vi "excelrowconcat_singlecol.vi"() -> ()   [LabVIEW 2020]
uses:
  <vilib>/addons/_office/excel.llb/Excel Get Data ([dbl]).vi
  <vilib>/Utility/file.llb/Write To Spreadsheet File (DBL).vi
  <vilib>/Utility/NIReport.llb/NI_report.lvclass
  <vilib>/Utility/NIReport.llb/Excel/NI_Excel.lvclass
  <vilib>/addons/_office/NI_ReportGenerationToolkit.lvlib
panel:
  out "LR Sheet Values":ext[][](array[numeric])=[[1.0, 16.0, 31.0, 46.0], [2.0, 17.0, 32.0, 47.0], [3.0, 18.0, 33.0, 48.0], [4.0, 19.0, 34.0, 49.0], [5.0, 20.0, 35.0, 50.0], [6.0, 21.0, 36.0, 51.0], [7.0, 22.0, 37.0, 52.0], [8.0, 23.0, 38.0, 53.0], [9.0, 24.0, 39.0, 54.0], [10.0, 25.0, 40.0, 55.0], [11.0, 26.0, 41.0, 56.0], [12.0, 27.0, 42.0, 57.0], [13.0, 28.0, 43.0, 58.0], [14.0, 29.0, 44.0, 59.0], [15.0, 30.0, 45.0, 60.0]] format="%_6e"
  out "Total LR Selected Row":i32=3
  in  "Tab Control":enum32{"HR", "LR"}(tab)
  out "LR Stack Col":ext[](array[numeric])=[1.0, 3.0, 5.0, 16.0, 18.0, 20.0, 31.0, 33.0, 35.0, 46.0, 48.0, 50.0] format="%#_6e"
  out "LR Added row":ext[][](array[numeric])=[[1.0, 16.0, 31.0, 46.0], [3.0, 18.0, 33.0, 48.0], [5.0, 20.0, 35.0, 50.0]] format="%#_6e"
  out "LR Selected Column":ext[](array[numeric])=[46.0, 48.0, 50.0] format="%#_6e"
  out "LR selected row":ext[](array[numeric])=[5.0, 20.0, 35.0, 50.0] format="%#_6e"
  in  "Low resgistananc state  Row Number (2,4,)":string="1,3,5"
  out "Columns":i32=4
  out "Rows":i32=15
  in  "Excel._Worksheet":refnum<k7>
  in  "Excel._Application":refnum<k7>
  out "HR Stack Col":ext[](array[numeric])=[1.0, 3.0, 5.0, 16.0, 18.0, 20.0, 31.0, 33.0, 35.0, 46.0, 48.0, 50.0] format="%#_6e"
  out "HR Selected Column":ext[](array[numeric])=[46.0, 48.0, 50.0] format="%#_6e"
  in  "precission":string="6"
  in  "Destination path for cutting rows":path=path "C:/Users/lab user/Desktop/cm/single column"
  in  "row cut file name (no extension)":string="saaaa"
  out "HR selected row":ext[](array[numeric])=[5.0, 20.0, 35.0, 50.0] format="%#_6e"
  in  "Hi resgistananc state  Row Number (1,3,)":string="1,3,5"
  out "Total HR Selected Row":i32=3
  in  "Select Excel file":path=path "C:/Users/lab user/Desktop/cm/single column/sc.xls"
  out "HR Added row":ext[][](array[numeric])=[[1.0, 16.0, 31.0, 46.0], [3.0, 18.0, 33.0, 48.0], [5.0, 20.0, 35.0, 50.0]] format="%#_6e"
  out "HR Sheet Values":ext[][](array[numeric])=[[1.0, 16.0, 31.0, 46.0], [2.0, 17.0, 32.0, 47.0], [3.0, 18.0, 33.0, 48.0], [4.0, 19.0, 34.0, 49.0], [5.0, 20.0, 35.0, 50.0], [6.0, 21.0, 36.0, 51.0], [7.0, 22.0, 37.0, 52.0], [8.0, 23.0, 38.0, 53.0], [9.0, 24.0, 39.0, 54.0], [10.0, 25.0, 40.0, 55.0], [11.0, 26.0, 41.0, 56.0], [12.0, 27.0, 42.0, 57.0], [13.0, 28.0, 43.0, 58.0], [14.0, 29.0, 44.0, 59.0], [15.0, 30.0, 45.0, 60.0]] format="%_6e"
  # "HR column stack output will be save in same directory\nrow cut file name_HR_single_col.xls"
  # "LR column stack output will be save in same directory\nrow cut file name_LR_single_col.xls"
  # "HR Row cut output will be save in same directory\nrow cut file name_HR.xls"
  # "LR Row cut  output will be save in same directory\nrow cut file name_LR.xls"
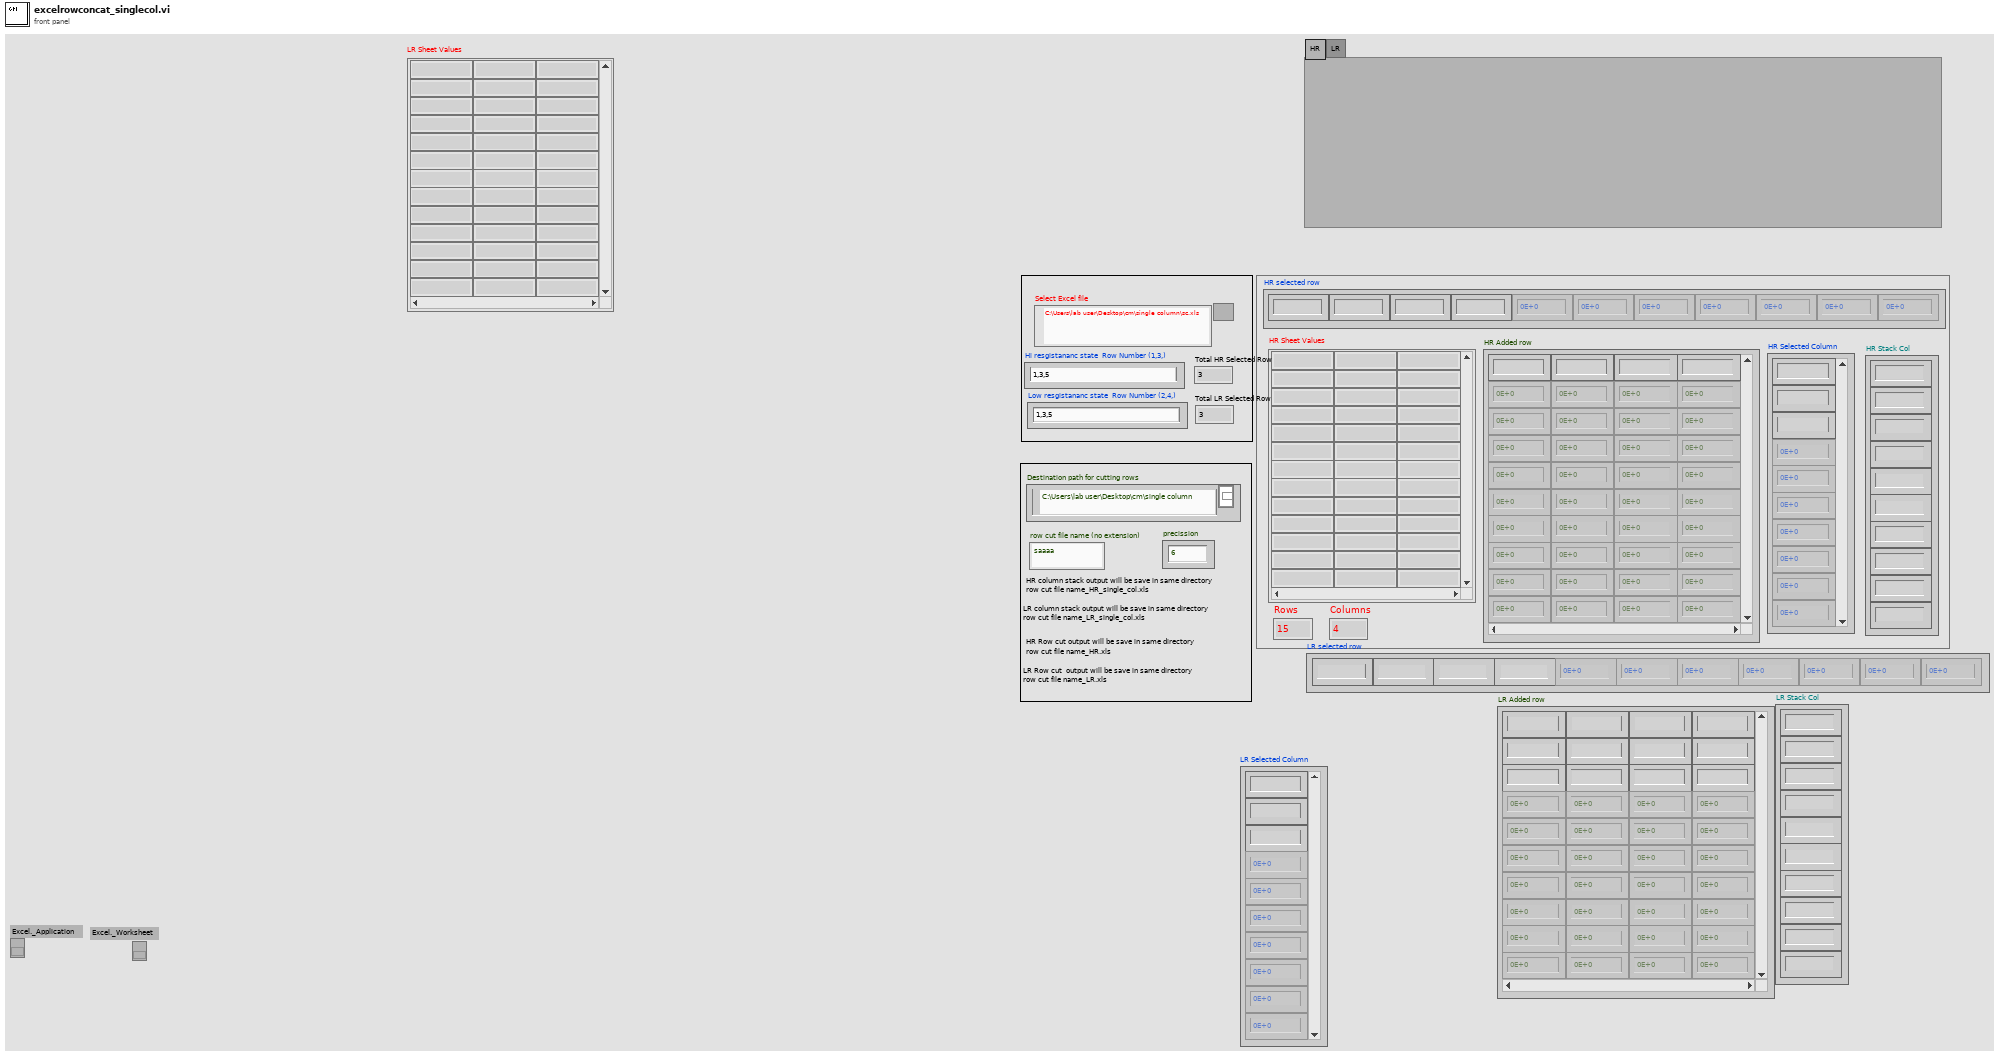
[diagram p1: front panel]
types:
  T1 = enum16{"Standard Report", "HTML", "Word", "Excel"}
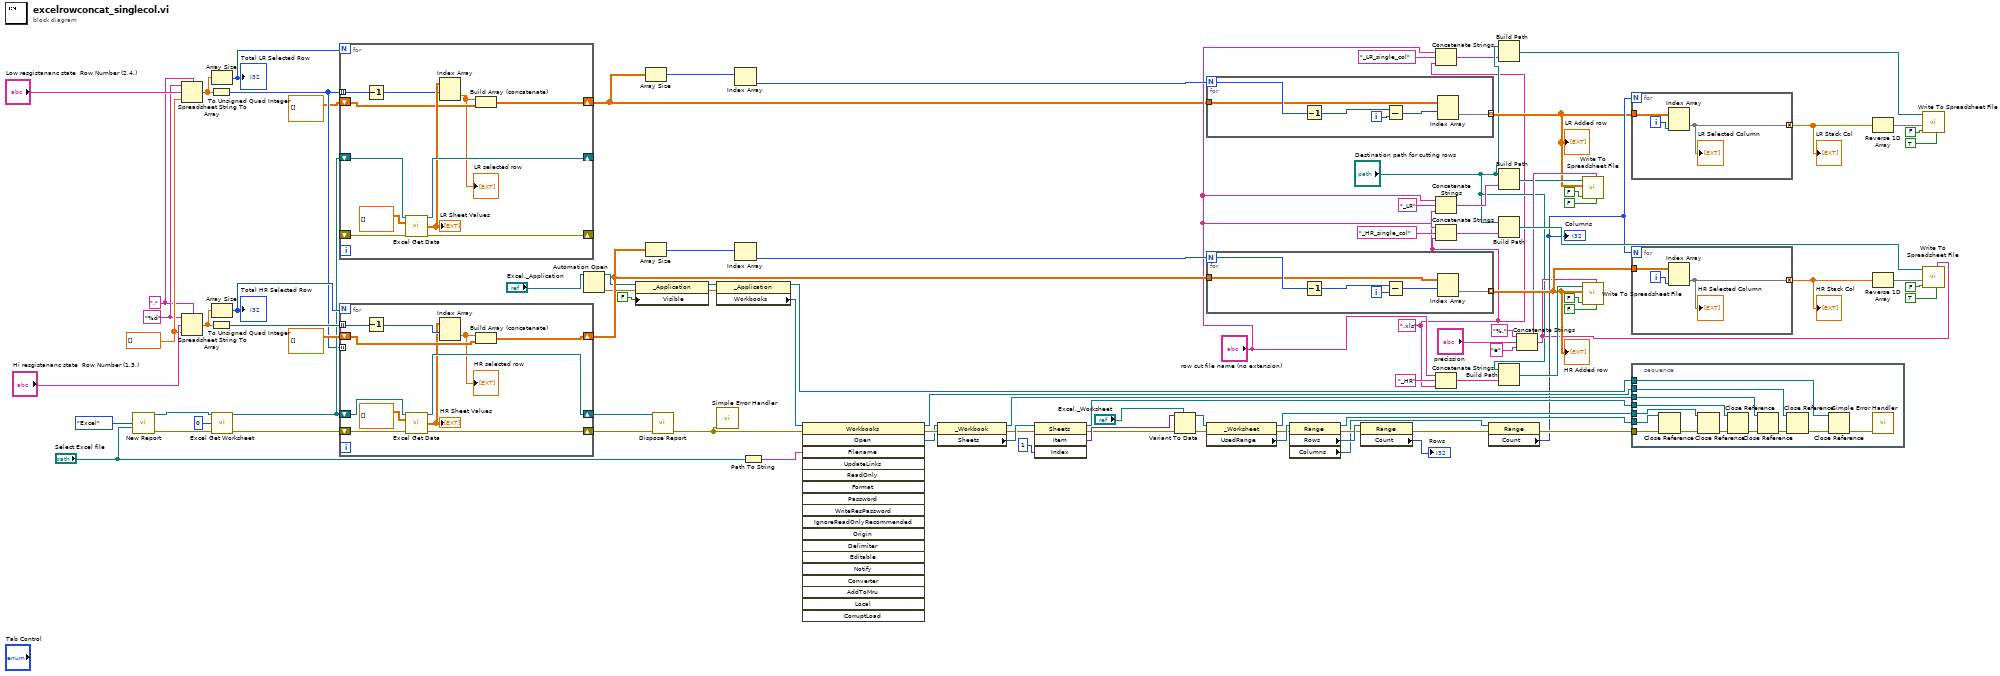
[diagram p0: block diagram]
diagram:
  w11 = ".xls" ("string")
  w32 = dbl[] []
  w29 = "," ("delimiter (Tab)")
  w30 = "%d" ("format string")
  n1 = call <vilib>:"New Report.vi"("report type"=T1."Excel", "template (empty)"="Select Excel file") -> ("report out"=w86:refnum<class "NI_report.lvclass">, "error out"=w87:errorcluster)  [unwired: 12 in]
  n2 = Spreadsheet String To Array(delimiter (Tab)=w29, format string=w30, spreadsheet string="Low resgistananc state  Row Number (2,4,)", array type (2D Dbl)=w32) -> (array=w6:dbl[])
  n3 = Spreadsheet String To Array(delimiter (Tab)=w29, format string=w30, spreadsheet string="Hi resgistananc state  Row Number (1,3,)", array type (2D Dbl)=w32) -> (array=w90:dbl[])
  n4 = To Unsigned Quad Integer(1:w6) -> (0:w4:u64[])
  n5 = To Unsigned Quad Integer(1:w90) -> (0:w89:u64[])
  n6 = Array Size(array=w6) -> (size(s)=w1:i32)
  "Total LR Selected Row" <- w1
  n7 = Array Size(array=w90) -> (size(s)=w69:i32)
  "Total HR Selected Row" <- w69
  n8 = call <vilib>:"Excel Get Worksheet.vi"("report in"=w86, "worksheet index (0)"=0, "error in (no error)"=w87) -> ("report out"=w5:refnum<class "NI_report.lvclass">, "error out"=w85:errorcluster)  [unwired: 11 in]
  n9 = for {
    N: w1 -> [_]
    shift-right: [w105] -> _
    shift-left: w5 -> [w102]
    shift-right: [w104] -> _
    shift-left: _ -> [w103]
    tunnel: w4 -> [w100] mode=indexing
    shift-right: [w98] -> w3
    shift-left: ext[][] [] -> [w97]
    n10 = Decrement(x=w100) -> (x-1=w99:u64)
    n11 = call-poly <vilib>:"Excel Get Data.vi"("report in"=w102, "data type"=ext[][] [], "error in (no error)"=w103) -> ("report out"=w105:refnum<class "NI_report.lvclass">, "data"=w101:ext[][], "error out"=w104:errorcluster)  [unwired: 10 in]
    "LR Sheet Values" <- w101
    n12 = Index Array(array=w101, index (row)=w99) -> (element=w96:ext[])  [unwired: 1 in]
    "LR selected row" <- w96
    n13 = Build Array (concatenate)(w96, w97) -> (w98:ext[][])
  }
  n14 = for {
    N: w69 -> [_]
    shift-right: [w116] -> w95
    shift-left: w5 -> [w111]
    shift-right: [w115] -> w94
    shift-left: w85 -> [w112]
    shift-right: [w113] -> w84
    shift-left: ext[][] [] -> [w114]
    tunnel: w89 -> [w110] mode=indexing
    tunnel: w4 -> [_] mode=indexing
    n15 = Decrement(x=w110) -> (x-1=w109:u64)
    n16 = call-poly <vilib>:"Excel Get Data.vi"("report in"=w111, "data type"=ext[][] [], "error in (no error)"=w112) -> ("report out"=w116:refnum<class "NI_report.lvclass">, "data"=w107:ext[][], "error out"=w115:errorcluster)  [unwired: 10 in]
    "HR Sheet Values" <- w107
    n17 = Index Array(array=w107, index (row)=w109) -> (element=w108:ext[])  [unwired: 1 in]
    "HR selected row" <- w108
    n18 = Build Array (concatenate)(w108, w114) -> (w113:ext[][])
  }
  n19 = Automation Open(Automation Refnum="Excel._Application") -> (Automation Refnum=w59:refnum<k7>, error out=w62:errorcluster)  [unwired: 3 in]
  n20 = property class="_Application"(reference=w59, error in=w62, "Visible"=FALSE ("Make Excel Visible")) -> (reference out=w58:refnum<k7>, error out=w61:errorcluster)
  n21 = Array Size(array=w3) -> (size(s)=w27:i32[])
  n22 = Array Size(array=w84) -> (size(s)=w82:i32[])
  n23 = call-dynamic "Dispose Report.vi"("report in"=w95, "error in (no error)"=w94) -> ("error out"=w35:errorcluster)  [unwired: 13 in]
  n24 = property class="_Application"(reference=w58, error in=w61) -> (reference out=w44:refnum<k7>, "Workbooks"=w47:refnum<k7>)  [unwired: 1 out]
  n25 = call <vilib>:"Simple Error Handler.vi"("error in (no error)"=w35) -> ()  [unwired: 4 in, 5 out]
  n26 = Index Array(array=w27) -> (element=w26:i32)  [unwired: 1 in]
  n27 = Index Array(array=w82) -> (element=w83:i32)  [unwired: 1 in]
  n28 = Path To String(path="Select Excel file") -> (string=w36:string)
  n29 = invoke class="Workbooks" method="Open"(reference=w47, error in=w35, "Filename"=w36) -> (reference out=w43:refnum<k7>, error out=w65:errorcluster, "Open"=w53:refnum<k7>)  [unwired: 15 in, 15 out]
  n30 = property class="_Workbook"(reference=w53, error in=w65) -> (reference out=w42:refnum<k7>, error out=w52:errorcluster, "Sheets"=w54:refnum<k7>)
  n31 = invoke class="Sheets" method="Item"(reference=w54, error in=w52, "Index"=1) -> (reference out=w41:refnum<k7>, error out=w51:errorcluster, "Item"=w64:variant)  [unwired: 1 in, 1 out]
  n32 = Variant To Data(error in=w51, type="Excel._Worksheet", Variant=w64) -> (data=w55:refnum<k7>, error out=w50:errorcluster)
  n33 = for {
    N: w26 -> [w123]
    tunnel: w3 -> [w120]
    tunnel: [w118] -> w16 mode=indexing
    i -> [w121]
    n34 = Decrement(x=w123) -> (x-1=w122:i32)
    n35 = Subtract(x=w122, y=w121) -> (x-y=w119:i32)
    n36 = Index Array(array=w120, index (row)=w119) -> (element=w118:ext[])  [unwired: 1 in]
  }
  "LR Added row" <- w16
  n37 = for {
    N: w83 -> [w129]
    tunnel: w84 -> [w126]
    tunnel: [w124] -> w75 mode=indexing
    i -> [w127]
    n38 = Decrement(x=w129) -> (x-1=w128:i32)
    n39 = Subtract(x=w128, y=w127) -> (x-y=w125:i32)
    n40 = Index Array(array=w126, index (row)=w125) -> (element=w124:ext[])  [unwired: 1 in]
  }
  "HR Added row" <- w75
  n41 = property class="_Worksheet"(reference=w55, error in=w50) -> (reference out=w40:refnum<k7>, error out=w49:errorcluster, "UsedRange"=w56:refnum<k7>)
  n42 = property class="Range"(reference=w56, error in=w49) -> (reference out=w39:refnum<k7>, error out=w48:errorcluster, "Rows"=w57:refnum<k7>, "Columns"=w45:refnum<k7>)
  n43 = property class="Range"(reference=w57, error in=w48) -> (error out=w38:errorcluster, "Count"=→"Rows":i32)  [unwired: 1 out]
  n44 = Concatenate Strings("row cut file name (no extension)", "_LR_single_col" ("string"), w11) -> (w9:string)
  n45 = Concatenate Strings("row cut file name (no extension)", "_LR" ("string"), w11) -> (w19:string)
  n46 = Concatenate Strings("row cut file name (no extension)", "_HR_single_col" ("string"), w11) -> (w70:string)
  n47 = Concatenate Strings("row cut file name (no extension)", "_HR" ("string"), w11) -> (w33:string)
  n48 = property class="Range"(reference=w45, error in=w38) -> (error out=w37:errorcluster, "Count"=w25:i32)  [unwired: 1 out]
  "Columns" <- w25
  n49 = Build Path(base path="Destination path for cutting rows", name or relative path=w9) -> (appended path=w8:path)
  n50 = Build Path(base path="Destination path for cutting rows", name or relative path=w19) -> (appended path=w17:path)
  n51 = Build Path(base path="Destination path for cutting rows", name or relative path=w70) -> (appended path=w72:path)
  n52 = Build Path(base path="Destination path for cutting rows", name or relative path=w33) -> (appended path=w79:path)
  n53 = Concatenate Strings("%.", "precission", "e") -> (w18:string)
  n54 = call-poly <vilib>:"Write To Spreadsheet File.vi"("transpose? (no:F)"=FALSE, "format (%.3f)"=w18, "append to file? (new file:F)"=FALSE, "2D data"=w16, "file path (dialog if empty)"=w17) -> ()  [unwired: 3 in, 1 out]
  n55 = call-poly <vilib>:"Write To Spreadsheet File.vi"("transpose? (no:F)"=FALSE, "format (%.3f)"=w18, "append to file? (new file:F)"=FALSE, "2D data"=w75, "file path (dialog if empty)"=w79) -> ()  [unwired: 3 in, 1 out]
  n56 = for {
    N: w25 -> [_]
    tunnel: w16 -> [w131]
    tunnel: [w130] -> w24 mode=concatenating
    i -> [w132]
    n57 = Index Array(array=w131, index (col)=w132) -> (element=w130:ext[])  [unwired: 1 in]
    "LR Selected Column" <- w130
  }
  "LR Stack Col" <- w24
  n58 = for {
    N: w25 -> [_]
    tunnel: w75 -> [w134]
    tunnel: [w133] -> w68 mode=concatenating
    i -> [w135]
    n59 = Index Array(array=w134, index (col)=w135) -> (element=w133:ext[])  [unwired: 1 in]
    "HR Selected Column" <- w133
  }
  "HR Stack Col" <- w68
  n60 = stacked-sequence {
    tunnel: w44 -> [w148]
    tunnel: w43 -> [w147]
    tunnel: w42 -> [w146]
    tunnel: w41 -> [w145]
    tunnel: w40 -> [w144]
    tunnel: w39 -> [w143]
    tunnel: w37 -> [w142]
    frame #0 {
      n61 = Close Reference(reference=w143, error in (no error)=w142) -> (error out=w141:errorcluster)
      n62 = Close Reference(reference=w144, error in (no error)=w141) -> (error out=w140:errorcluster)
      n63 = Close Reference(reference=w145, error in (no error)=w140) -> (error out=w139:errorcluster)
      n64 = Close Reference(reference=w146, error in (no error)=w139) -> (error out=w138:errorcluster)
      n65 = Close Reference(reference=w147, error in (no error)=w138) -> (error out=w137:errorcluster)
      n66 = Close Reference(reference=w148, error in (no error)=w137) -> (error out=w136:errorcluster)
      n67 = call <vilib>:"Simple Error Handler.vi"("error in (no error)"=w136) -> ()  [unwired: 4 in, 5 out]
    }
  }
  n68 = Reverse 1D Array(array=w24) -> (reversed array=w7:ext[])
  n69 = Reverse 1D Array(array=w68) -> (reversed array=w67:ext[])
  n70 = call-poly <vilib>:"Write To Spreadsheet File.vi"("transpose? (no:F)"=TRUE, "append to file? (new file:F)"=FALSE, "1D data"=w7, "file path (dialog if empty)"=w8) -> ()  [unwired: 4 in, 1 out]
  n71 = call-poly <vilib>:"Write To Spreadsheet File.vi"("transpose? (no:F)"=TRUE, "format (%.3f)"=w18, "append to file? (new file:F)"=FALSE, "1D data"=w67, "file path (dialog if empty)"=w72) -> ()  [unwired: 3 in, 1 out]
